vi "Final.vi"() -> ()   [LabVIEW 2014]
uses:
  <vilib>/sound2/lvsound2.llb/Sound Data Format.ctl
  <vilib>/sound2/lvsound2.llb/Sampling Mode.ctl
  <vilib>/event_ctls.llb/eventvkey.ctl
  <vilib>/sound2/lvsound2.llb/Sound Output Write (DBL Single).vi
  <vilib>/measure/NI_MABase.lvlib
panel:
  in  "Automatic notes":string="E4 E4 ~ E4 ~ C4 E4 ~ G4 ~ ~ ~ G3 ~ ~ ~ C4 ~ ~ G3 ~ ~ E3 ~ ~ A3 ~ B3 ~ A3# A3 ~ G3 E4 G4 A4 ~ F4 ~ G4 ~ E4 ~ C4 D4 B3 ~ ~ C4 ~ ~ G3 ~ ~ E3 ~ ~ A3 ~ B3 ~ A3# A3 ~ G3 E4 G4 A4 ~ F4 ~ G4 ~ E4 ~ C4 D4 B3 ~ ~ ~ ~ G4 F4# F4 D4# ~ E4 ~ G3 A3 C4 ~ A3 C4 D4 ~ ~ G4 F4# F4 D4# ~ E4 ~ C5 ~ C5 C5 ~ ~ ~ ~ ~ G4 F4# F4 D4# ~ E4 ~ G3 A3 C4 ~ A3 C4 D4 ~ ~ D4# ~ ~ D4 ~ ~ C4 "
  in  "Valid Notes":T1(ring)
  out "Frequency":dbl
  in  "stop":bool
  in  "mode":bool
  in  "Piano":T2
  # "輸入設定好的程式碼後，執行會自動撥放程式碼對應到的音色。"
  # "選擇模式後執行"
  # "顯示對應到的頻率"
  # "鍵盤輸入:\na → C4\nw → C4#\ns → D4\ne → D4#\nd → E4\nf → F4\nt → F4#\ng → G4\ny → G4#\nh → A4\nu → A4#\nj → B4\nk → C5"
  # "可用鍵盤輸入或用滑鼠輸入輸出對應到的音色，按stop結束程式。"
  # "C4"
  # "C3"
  # "C5"
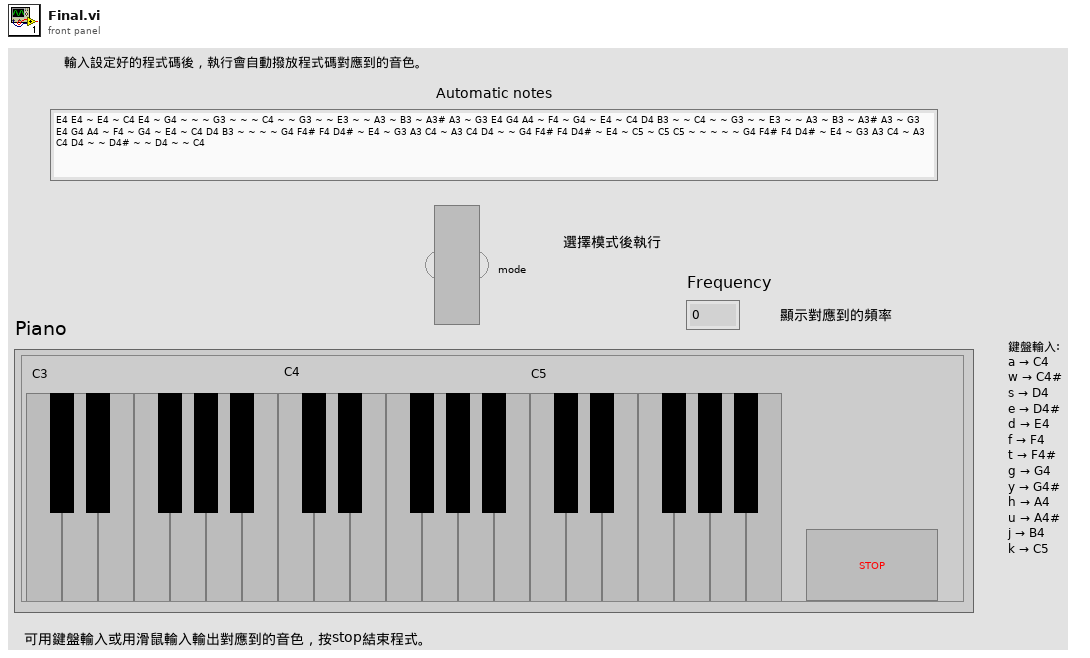
[diagram p1: front panel]
types:
  T1 = enum16{"~", "C1", "C1#", "D1", "D1#", "E1", "F1", "F1#", "G1", "G1#", "A1", "A1#", "B1", "C2", "C2#", "D2", "D2#", "E2", "F2", "F2#", "G2", "G2#", "A2", "A2#", "B2", "C3", "C3#", "D3", "D3#", "E3", "F3", "F3#", "G3", "G3#", "A3", "A3#", "B3", "C4", "C4#", "D4", "D4#", "E4", "F4", "F4#", "G4", "G4#", "A4", "A4#", "B4", "C5", "C5#", "D5", "D5#", "E5", "F5", "F5#", "G5", "G5#", "A5", "A5#", "B5", "C6", "C6#", "D6", "D6#", "E6", "F6", "F6#", "G6", "G6#", "A6", "A6#", "B6", "C7", "C7#", "D7", "D7#", "E7", "F7", "F7#", "G7", "G7#", "A7", "A7#", "B7", "C8", ""}
  T2 = cluster{"C3":bool, "C3#":bool, "D3":bool, "D3#":bool, "E3\nE3":bool, "F3":bool, "F3#":bool, "G3":bool, "G3#":bool, "A3":bool, "A3#":bool, "B3":bool, "C4":bool, "C4#":bool, "D4":bool, "D4#":bool, "E4":bool, "F4":bool, "F4#":bool, "G4\nG4":bool, "G4#":bool, "A4":bool, "A4#":bool, "B4":bool, "C5":bool, "C5#":bool, "D5":bool, "D5#":bool, "E5":bool, "F5":bool, "F5#":bool, "G5\nG4 2":bool, "G5#":bool, "A5":bool, "A5#":bool, "B5":bool}
  T3 = typedef "Sampling Mode.ctl" = i32
  T4 = typedef "Sound Data Format.ctl" = cluster{"sample rate (S/s)":dbl, "number of channels":i32, "bits per sample":i32}
  T5 = typedef "Sound Output Task ID.ctl" = u32
  T6 = typedef "eventvkey.ctl" = enum16{"ASCII", "Enter", "Return", "Shift", "Ctrl", "Alt", "Cmd", "Opt", "Caps", "NumLock", "Clear", "Break", "Up", "Down", "Left", "Right", "Insert", "Delete", "Home", "End", "PageUp", "PageDown", "Escape", "Help", "Pause", "ScrollLock", "F1", "F2", "F3", "F4", "F5", "F6", "F7", "F8", "F9", "F10", "F11", "F12", "F13", "F14", "F15", "F16", "F17", "F18", "F19", "F20", "F21", "F22", "F23", "F24", "Play", "VolumeUp", "VolumeDown", "Mute", "Two Byte Char"}
  T7 = cluster{"[0]":bool, "[1]":bool, "[2]":bool, "[3]":bool, "[4]":bool, "[5]":bool, "[6]":bool, "[7]":bool, "[8]":bool, "[9]":bool, "[10]":bool, "[11]":bool, "[12]":bool, "[13]":bool, "[14]":bool, "[15]":bool, "[16]":bool, "[17]":bool, "[18]":bool, "[19]":bool, "[20]":bool, "[21]":bool, "[22]":bool, "[23]":bool, "[24]":bool, "[25]":bool, "[26]":bool, "[27]":bool, "[28]":bool, "[29]":bool, "[30]":bool, "[31]":bool, "[32]":bool, "[33]":bool, "[34]":bool, "[35]":bool}
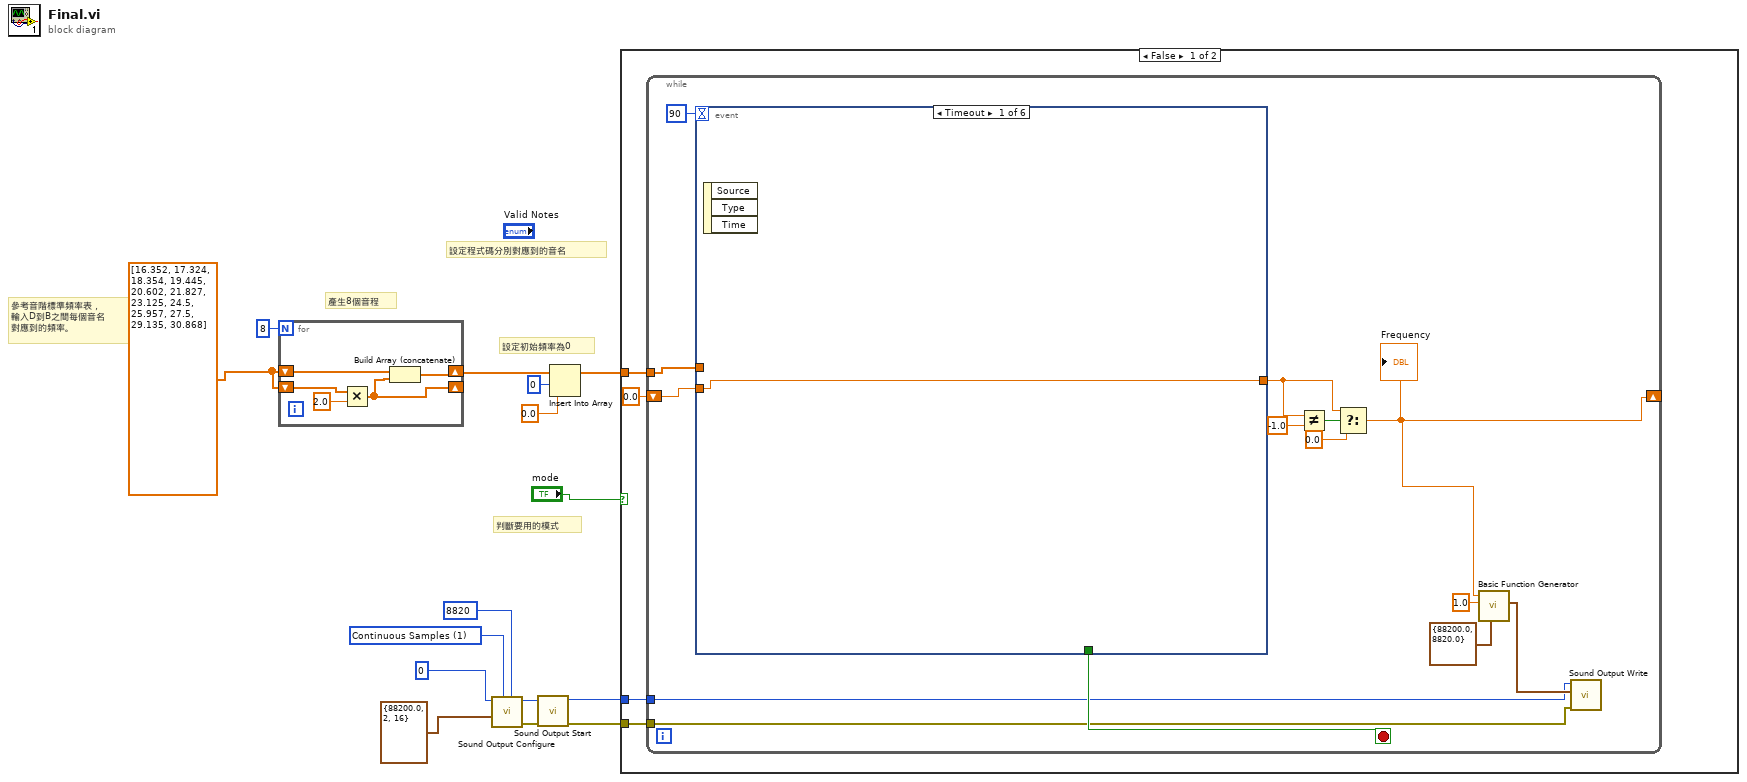
[diagram p0: block diagram]
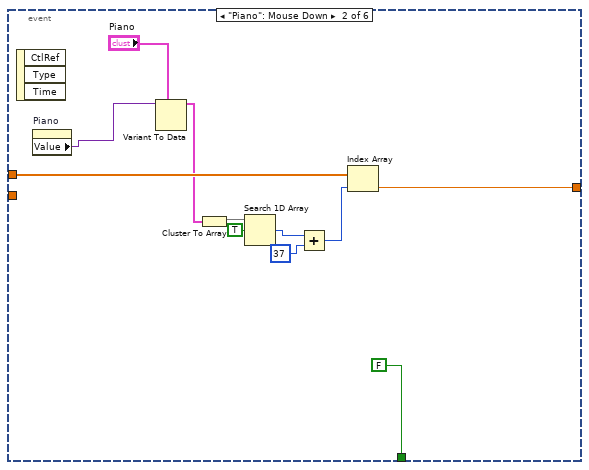
[diagram p2: hidden frame]
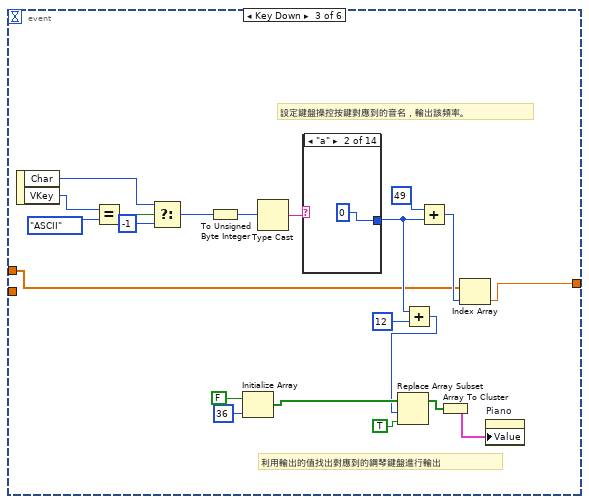
[diagram p3: hidden frame]
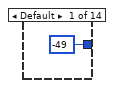
[diagram p4: hidden frame]
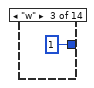
[diagram p5: hidden frame]
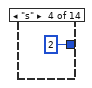
[diagram p6: hidden frame]
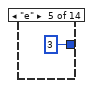
[diagram p7: hidden frame]
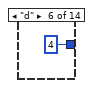
[diagram p8: hidden frame]
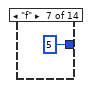
[diagram p9: hidden frame]
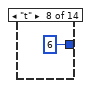
[diagram p10: hidden frame]
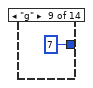
[diagram p11: hidden frame]
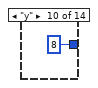
[diagram p12: hidden frame]
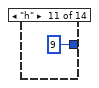
[diagram p13: hidden frame]
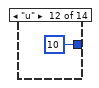
[diagram p14: hidden frame]
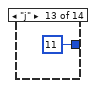
[diagram p15: hidden frame]
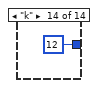
[diagram p16: hidden frame]
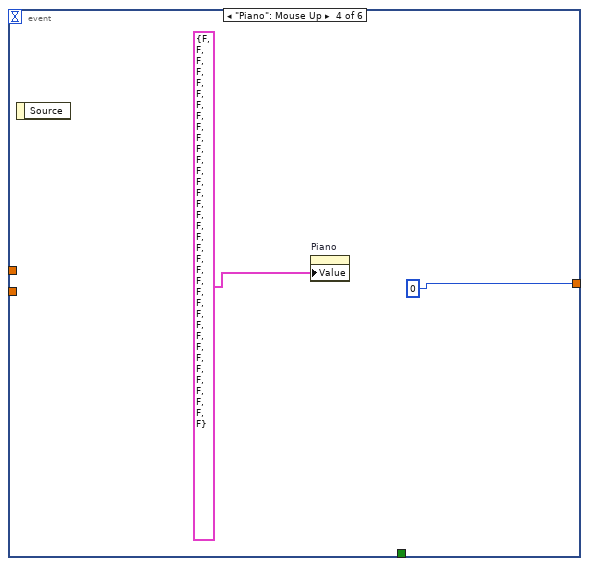
[diagram p17: hidden frame]
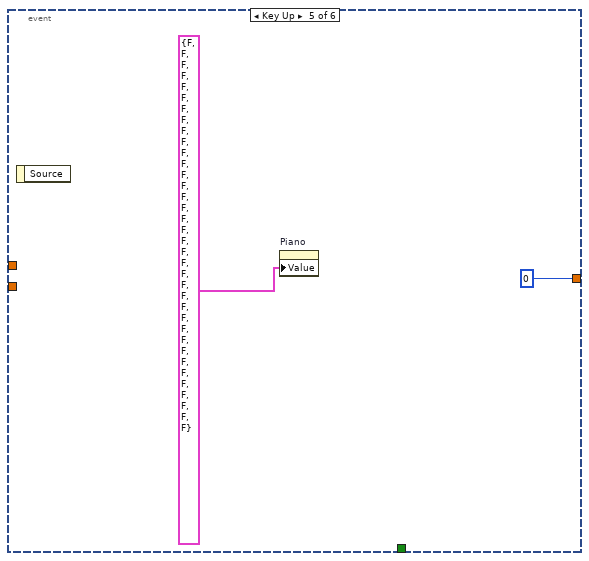
[diagram p18: hidden frame]
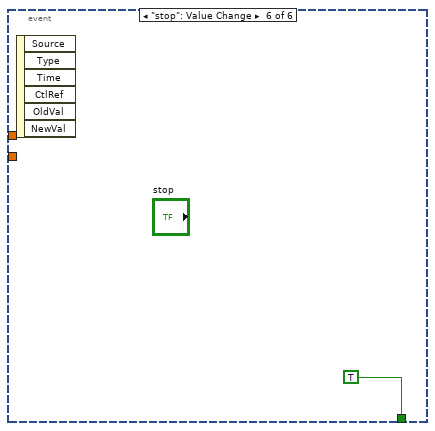
[diagram p19: hidden frame]
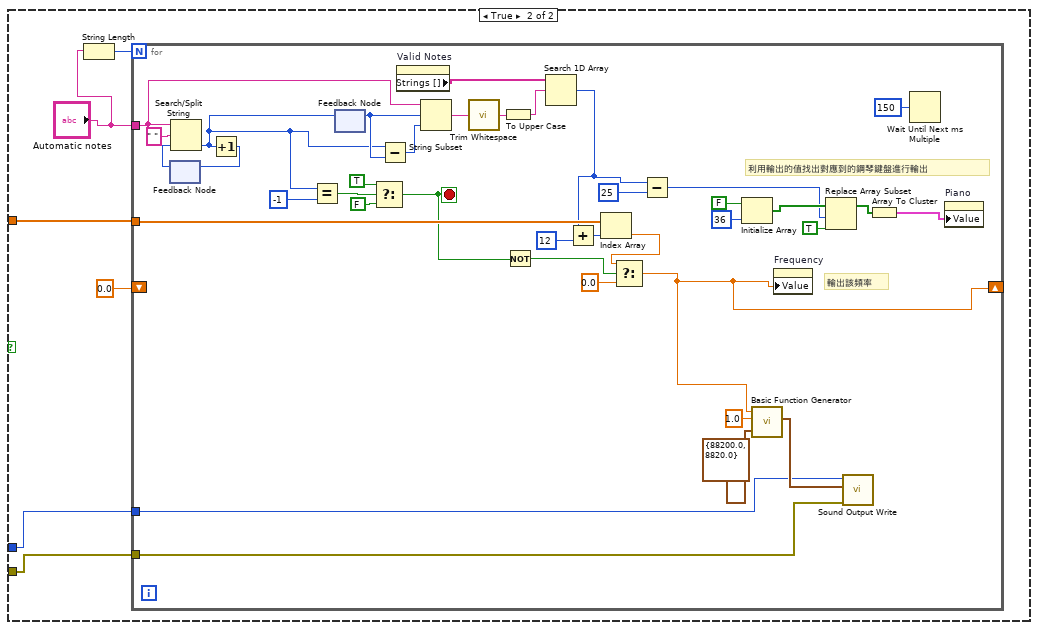
[diagram p20: hidden frame]
diagram:
  w4 = T3 1 items=["Finite Samples", "Continuous Samples"] ("sample mode")
  w14 = dbl[] [16.352, 17.324, 18.354, 19.445, 20.602, 21.827, 23.125, 24.5, 25.957, 27.5, 29.135, 30.868]
  # "判斷要用的模式"
  # "設定程式碼分別對應到的音名"
  # "設定初始頻率為0"
  # "產生8個音程"
  # "參考音階標準頻率表，\n輸入D到B之間每個音名\n對應到的頻率。"
  n1 = for {
    N: 8 -> [_]
    shift-right: [w17] -> w13
    shift-left: w14 -> [w18]
    shift-right: [w16] -> _
    shift-left: w14 -> [w19]
    n2 = Multiply(x=w19, y=2.0) -> (x*y=w16:dbl[])
    n3 = Build Array (concatenate)(w18, w16) -> (w17:dbl[])
  }
  n4 = call <vilib>:"Sound Output Configure.vi"("number of samples/ch"=8820, "sample mode"=w4, "sound format"=T4 {"sample rate (S/s)"=88200.0, "number of channels"=2, "bits per sample"=16}, "device ID"=u32 0) -> ("error out"=w7:errorcluster, "task ID"=w8:T5)  [unwired: 6 in]
  n5 = call <vilib>:"Sound Output Start.vi"("error in (no error)"=w7, "task ID"=w8) -> ("error out"=w1:errorcluster, "task ID out"=w2:T5)  [unwired: 8 in]
  n6 = Insert Into Array(array=w13, index=0, new element=0.0 ("new element/subarray")) -> (w9:dbl[])
  n7 = case shown="False" "mode" {
    tunnel: w9 -> [w24 w94]
    tunnel: w2 -> [w22 w96]
    tunnel: w1 -> [w21 w95]
    frame False {
      n8 = while {
        tunnel: w24 -> [w38]
        shift-right: [w27] -> _
        shift-left: 0.0 ("f") -> [w33]
        tunnel: w22 -> [w26]
        tunnel: w21 -> [w25]
        stop <- w32 stop-if-true
        n9 = event shown="[0] Timeout" {
          selector: _ -> [_ _ _ _ _ _]
          dyn-events: _ -> [_ _ _ _ _ _]
          timeout: 90 -> [_ _ _ _ _ _]
          tunnel: w38 -> [_ w49 w53 _ _ _]
          tunnel: [w39 w42 w59 0 0 _] -> w35
          tunnel: w33 -> [w39 _ _ _ _ _]
          tunnel: [_ FALSE _ _ _ TRUE] -> w32
          event Timeout {
            n10 = event-data() -> ()  [unwired: 1 in, 3 out]
          }
          event "Piano": Mouse Down {
            n11 = event-data() -> ()  [unwired: 1 in, 3 out]
            n12 = property on="Piano" class="Clust"() -> ("Value"=w40:variant)  [unwired: 2 in, 2 out]
            n13 = Variant To Data(type="Piano", Variant=w40) -> (data=w48:T2)  [unwired: 1 in, 1 out]
            n14 = Cluster To Array(cluster=w48) -> (array=w47:bool[])
            n15 = Search 1D Array(1D array=w47, element=TRUE) -> (index of element=w45:i32)  [unwired: 1 in]
            n16 = Add(x=w45, y=37) -> (x+y=w43:i32)
            n17 = Index Array(array=w49, index=w43) -> (element=w42:dbl)
          }
          event Key Down {
            # "利用輸出的值找出對應到的鋼琴鍵盤進行輸出"
            # "設定鍵盤操控按鍵對應到的音名，輸出該頻率。"
            n18 = event-data() -> ("Char"=w68:i16, "VKey"=w71:T6)  [unwired: 1 in]
            n19 = Equal?(x=w71, y=eventvkey."ASCII") -> (x = y?=w69:bool)
            n20 = Select(t=w68, s=w69, f=i16 -1) -> (s? t:f=w66:i16)
            n21 = To Unsigned Byte Integer(number=w66) -> (unsigned 8bit integer=w65:u8)
            n22 = Initialize Array(FALSE, 36 ("dimension size")) -> (w56:bool[])
            n23 = Type Cast(x=w65) -> (*(type *) &x=w64:string)  [unwired: 1 in]
            n24 = case shown="\"a\"" w64 {
              tunnel: [-49 0 1 2 3 4 5 6 7 8 9 10 11 12] -> w58
              frame Default {
              }
              frame "a" {
              }
              frame "w" {
              }
              frame "s" {
              }
              frame "e" {
              }
              frame "d" {
              }
              frame "f" {
              }
              frame "t" {
              }
              frame "g" {
              }
              frame "y" {
              }
              frame "h" {
              }
              frame "u" {
              }
              frame "j" {
              }
              frame "k" {
              }
            }
            n25 = Add(x=w58, y=12) -> (x+y=w55:i32)
            n26 = Replace Array Subset(array=w56, new element=TRUE, index=w55) -> (w51:bool[])
            n27 = Add(x=49, y=w58) -> (x+y=w60:i32)
            n28 = Array To Cluster(array=w51) -> (cluster=w52:T7)
            n29 = Index Array(array=w53, index=w60) -> (element=w59:dbl)
            n30 = property on="Piano" class="Clust"("Value"=w52) -> ()  [unwired: 2 in, 2 out]
          }
          event "Piano": Mouse Up {
            n31 = event-data() -> ()  [unwired: 1 in, 1 out]
            n32 = property on="Piano" class="Clust"("Value"=T2 {"C3"=FALSE, "C3#"=FALSE, "D3"=FALSE, "D3#"=FALSE, "E3\nE3"=FALSE, "F3"=FALSE, "F3#"=FALSE, "G3"=FALSE, "G3#"=FALSE, "A3"=FALSE, "A3#"=FALSE, "B3"=FALSE, "C4"=FALSE, "C4#"=FALSE, "D4"=FALSE, "D4#"=FALSE, "E4"=FALSE, "F4"=FALSE, "F4#"=FALSE, "G4\nG4"=FALSE, "G4#"=FALSE, "A4"=FALSE, "A4#"=FALSE, "B4"=FALSE, "C5"=FALSE, "C5#"=FALSE, "D5"=FALSE, "D5#"=FALSE, "E5"=FALSE, "F5"=FALSE, "F5#"=FALSE, "G5\nG4 2"=FALSE, "G5#"=FALSE, "A5"=FALSE, "A5#"=FALSE, "B5"=FALSE} ("Cluster")) -> ()  [unwired: 2 in, 2 out]
          }
          event Key Up {
            n33 = event-data() -> ()  [unwired: 1 in, 1 out]
            n34 = property on="Piano" class="Clust"("Value"=T2 {"C3"=FALSE, "C3#"=FALSE, "D3"=FALSE, "D3#"=FALSE, "E3\nE3"=FALSE, "F3"=FALSE, "F3#"=FALSE, "G3"=FALSE, "G3#"=FALSE, "A3"=FALSE, "A3#"=FALSE, "B3"=FALSE, "C4"=FALSE, "C4#"=FALSE, "D4"=FALSE, "D4#"=FALSE, "E4"=FALSE, "F4"=FALSE, "F4#"=FALSE, "G4\nG4"=FALSE, "G4#"=FALSE, "A4"=FALSE, "A4#"=FALSE, "B4"=FALSE, "C5"=FALSE, "C5#"=FALSE, "D5"=FALSE, "D5#"=FALSE, "E5"=FALSE, "F5"=FALSE, "F5#"=FALSE, "G5\nG4 2"=FALSE, "G5#"=FALSE, "A5"=FALSE, "A5#"=FALSE, "B5"=FALSE} ("Cluster")) -> ()  [unwired: 2 in, 2 out]
          }
          event "stop": Value Change {
            n35 = event-data() -> ()  [unwired: 1 in, 6 out]
          }
        }
        n36 = Not Equal?(x=w35, y=-1.0) -> (x != y?=w37:bool)
        n37 = Select(t=w35, s=w37, f=0.0) -> (s? t:f=w27:dbl)
        "Frequency" <- w27
        n38 = call <vilib>:"Basic Function Generator.vi"("sampling info"=cluster{"Fs":dbl, "#s":dbl} {"Fs"=88200.0, "#s"=8820.0}, "amplitude"=1.0, "frequency"=w27) -> ("signal out"=w28:waveform(dbl))  [unwired: 6 in, 2 out]
        n39 = call-poly <vilib>:"Sound Output Write.vi"("error in (no error)"=w25, "data"=w28, "task ID"=w26) -> ()  [unwired: 7 in, 2 out]
      }
    }
    frame True {
      n40 = String Length(string="Automatic notes") -> (length=w93:i32)
      n41 = for {
        N: w93 -> [_]
        tunnel: "Automatic notes" -> [w124]
        tunnel: w94 -> [w123]
        tunnel: w96 -> [w105]
        tunnel: w95 -> [w104]
        shift-right: [w97] -> _
        shift-left: 0.0 -> [_]
        stop <- w117 stop-if-true
        # "輸出該頻率"
        # "利用輸出的值找出對應到的鋼琴鍵盤進行輸出"
        n42 = feedback #1() -> (w132:i32)  [unwired: 1 in]
        n43 = Search/Split String(string=w124, search string/char (-)=" ", offset (0)=w132) -> (offset of match=w126:i32)  [unwired: 2 out]
        n44 = Increment(x=w126) -> (x+1=w133:i32)
        n45 = feedback-in #1(w133) -> ()
        n46 = Equal?(x=w126, y=-1) -> (x = y?=w130:bool)
        n47 = feedback-in #2(w126) -> ()
        n48 = feedback #2() -> (w127:i32)  [unwired: 1 in]
        n49 = Select(t=TRUE, s=w130, f=FALSE) -> (s? t:f=w117:bool)
        n50 = Subtract(x=w126, y=w127) -> (x-y=w125:i32)
        n51 = property on="Valid Notes" class="Enum (strict)"() -> ("Strings []"=w102:string[])  [unwired: 2 in, 2 out]
        n52 = String Subset(string=w124, offset (0)=w127, length (rest)=w125) -> (substring=w122:string)
        n53 = call <vilib>:"Trim Whitespace.vi"("string"=w122) -> ("trimmed string"=w121:string)  [unwired: 1 in]
        n54 = To Upper Case(1:w121) -> (0:w120:string)
        n55 = Not(x=w117) -> (.not. x?=w116:bool)
        n56 = Search 1D Array(1D array=w102, element=w120) -> (index of element=w99:i32)  [unwired: 1 in]
        n57 = Add(x=w99, y=12) -> (x+y=w100:i32)
        n58 = Index Array(array=w123, index=w100) -> (element=w119:dbl)
        n59 = Select(t=w119, s=w116, f=0.0) -> (s? t:f=w97:dbl)
        n60 = Subtract(x=w99, y=25) -> (x-y=w109:i32)
        n61 = Initialize Array(FALSE, 36 ("dimension size")) -> (w110:bool[])
        n62 = call <vilib>:"Basic Function Generator.vi"("sampling info"=cluster{"Fs":dbl, "#s":dbl} {"Fs"=88200.0, "#s"=8820.0}, "amplitude"=1.0, "frequency"=w97) -> ("signal out"=w106:waveform(dbl))  [unwired: 6 in, 2 out]
        n63 = property on="Frequency" class="DigNum (strict)"("Value"=w97) -> ()  [unwired: 2 in, 2 out]
        n64 = Replace Array Subset(array=w110, new element=TRUE, index=w109) -> (w113:bool[])
        n65 = call-poly <vilib>:"Sound Output Write.vi"("error in (no error)"=w104, "data"=w106, "task ID"=w105) -> ()  [unwired: 7 in, 2 out]
        n66 = Array To Cluster(array=w113) -> (cluster=w101:T7)
        n67 = Wait Until Next ms Multiple(millisecond multiple=u32 150) -> ()  [unwired: 1 out]
        n68 = property on="Piano" class="Clust"("Value"=w101) -> ()  [unwired: 2 in, 2 out]
      }
    }
  }
